vi "LJUD_Close.vi"(8 "error in":errorcluster) -> (0 "error out":errorcluster)   [LabVIEW 2021]
doc: "Closes all handles to all UD devices."
uses:
  labjackud.dll
panel:
  # "Closes all handles to all UD devices."
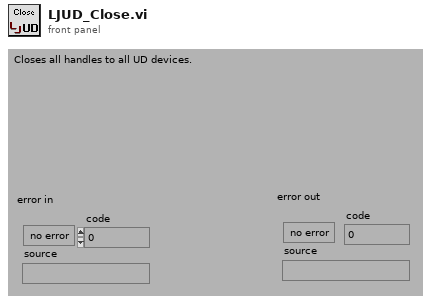
[diagram p1: front panel]
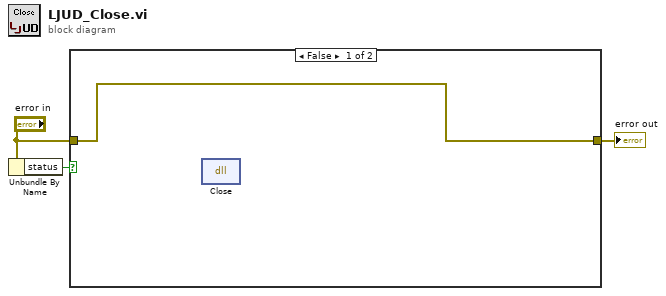
[diagram p0: block diagram]
diagram:
  n1 = Unbundle By Name("error in") -> ("status"=w2:bool)
  n2 = case shown="False" w2 {
    tunnel: [w4 w5] -> w3
    tunnel: "error in" -> [w4 w5]
    frame False {
      n3 = dll-call lib="labjackud.dll" fn="Close"() -> ()  [unwired: 4 in, 2 out]
    }
    frame True {
    }
  }
  "error out" <- w3
